vi "Autonomous Independent.vi"() -> ()   [LabVIEW 2020]
doc: "This VI is called when autonomous begins, and will automatically be terminated when autonomous ends. You can carry out timed or sensor driven robot movement independently without needing to return to the caller."
uses:
  <vilib>/Rock Robotics/WPI/Utilities/WPI_GetSetVariantRefNum.vi
  <vilib>/Rock Robotics/Network Tables/NT Read String.vi
  <vilib>/Rock Robotics/Network Tables/NT Write Numeric Array.vi
  <vilib>/Rock Robotics/WPI/RobotDrive/WPI_RobotDriveArcadeDrive_Standard(NoSaturation).vi
  2017 Swerve Code/Swerve Global Variables.vi
  Robot Global Data.vi
panel:
  out "Current Movement, for debugging":T1 {"Y Joystick Value" scale=1.0..-1.0; "X Joystick Value" scale=-1.0..1.0}
  in  "Array of robot movements":T2(array[cluster])=[{"X Joystick Value"=0.39393939393939403, "Y Joystick Value"=0.0, "Delay (sec)"=1.0, "Movement Name"="turn"}, {"X Joystick Value"=-0.3737373737373737, "Y Joystick Value"=0.0, "Delay (sec)"=1.0, "Movement Name"="turn back"}] {"Y Joystick Value" scale=1.0..-1.0; "X Joystick Value" scale=-1.0..1.0}
  # "Be sure to right-click and choose Data Operations>>Make Current Value default if you want to save the array values with the VI"
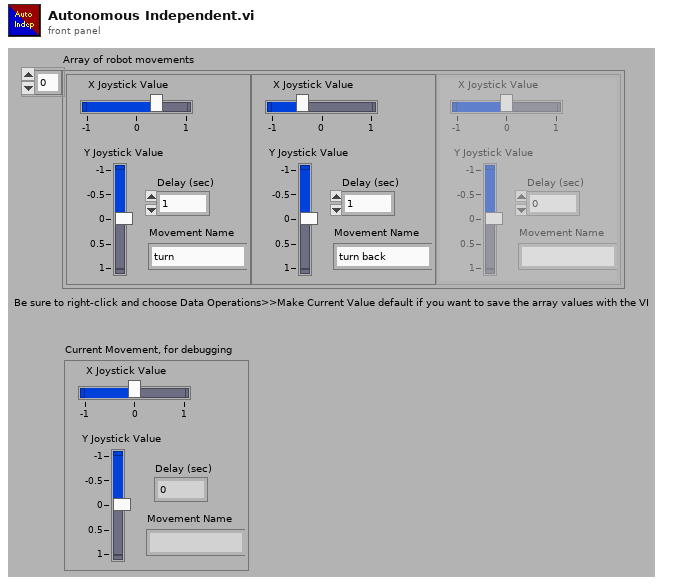
[diagram p1: front panel]
types:
  T1 = cluster{"X Joystick Value":dbl, "Y Joystick Value":dbl, "Delay (sec)":dbl, "Movement Name":string}
  T2 = cluster{"X Joystick Value":dbl, "Y Joystick Value":dbl, "Delay (sec)":dbl, "Movement Name":string}[]
  T3 = typedef "WPI_JoystickDevRef.ctl" = cluster{"Device":T4}
  T4 = typedef "WPI_JoystickDeviceEnum.ctl" = enum16{"USB 0", "USB 1", "USB 2", "USB 3", "USB 4", "USB 5"}
  T5 = typedef "WPI_RobotDriveDevRef.ctl" = cluster{"DevStatus":errorcluster, "Motors[]":T6[], "Square Inputs":bool, "Max Output":dbl}
  T6 = typedef "WPI_MotorControlDeviceRef.ctl" = cluster{"DeviceStatus":errorcluster, "Type":T7, "PWM":cluster{"PWM Channel":T8, "DeadBand":T9}, "CAN":cluster{"Device Number":u8, "SetOutput VI Ref":variant, "GetOutput VI Ref":variant, "Enable VI Ref":variant, "Disable VI Ref":variant, "Data":variant}, "Invert":bool, "DIO PWM":cluster{"PWM \"Enable\" Channel":T8, "DIOChannel":T10, "PWM Rate":dbl}}
  T7 = typedef "WPI_MotorControlType.ctl" = enum16{"PWM", "CAN", "DIO PWM"}
  T8 = typedef "FPGA_DIOPWMChannel.ctl" = enum8{"PWM 0", "PWM 1", "PWM 2", "PWM 3", "PWM 4", "PWM 5", "PWM 6", "PWM 7", "PWM 8", "PWM 9", "PWM MXP 0", "PWM MXP 1", "PWM MXP 2", "PWM MXP 3", "PWM MXP 4", "PWM MXP 5", "PWM MXP 6", "PWM MXP 7", "PWM MXP 8", "PWM MXP 9", "Invalid"}
  T9 = typedef "WPI_PWMDeadband.ctl" = cluster{"Name":string, "maxPositivePwm":i32, "minPositivePwm":i32, "centerPwm":i32, "maxNegativePwm":i32, "minNegativePwm":i32, "angularRange":u16}
  T10 = typedef "FPGA_DIOChannel.ctl" = enum8{"DIO 0", "DIO 1", "DIO 2", "DIO 3", "DIO 4", "DIO 5", "DIO 6", "DIO 7", "DIO 8", "DIO 9", "DIO MXP 0", "DIO MXP 1", "DIO MXP 2", "DIO MXP 3", "DIO MXP 4", "DIO MXP 5", "DIO MXP 6", "DIO MXP 7", "DIO MXP 8", "DIO MXP 9", "DIO MXP 10", "DIO MXP 11", "DIO MXP 12", "DIO MXP 13", "DIO MXP 14", "DIO MXP 15", "SPI Port CS1", "SPI Port CS2", "SPI Port CS3", "SPI Port MISO", "SPI Port MOSI", "Invalid"}
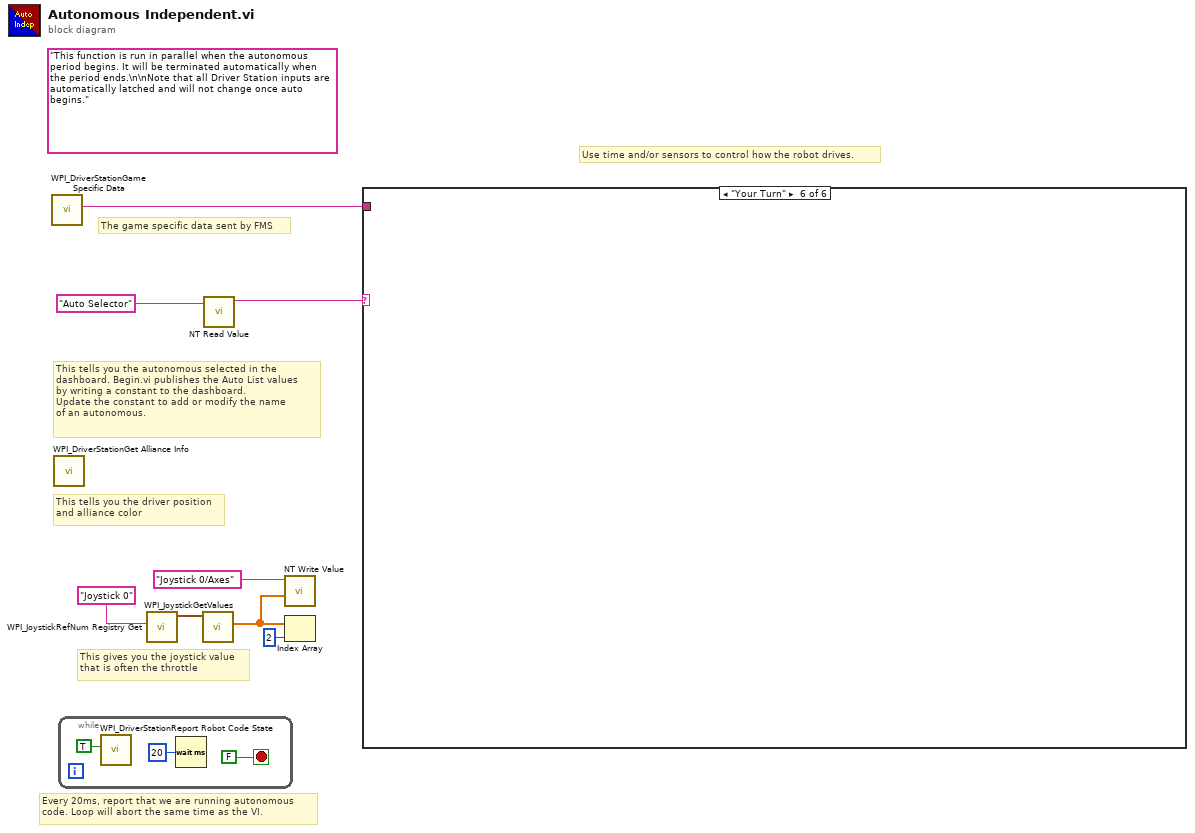
[diagram p0: block diagram]
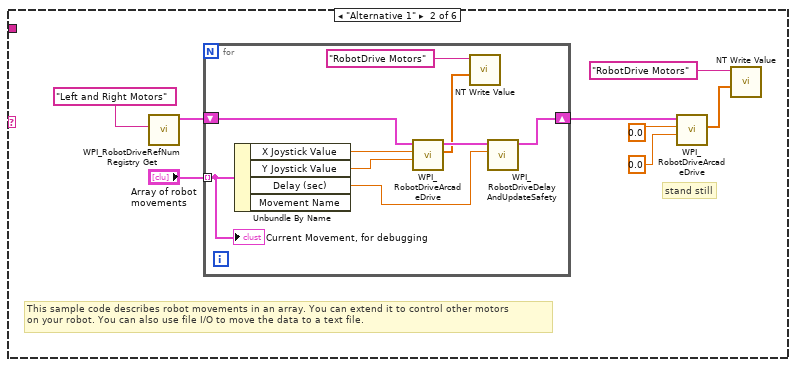
[diagram p3: hidden frame]
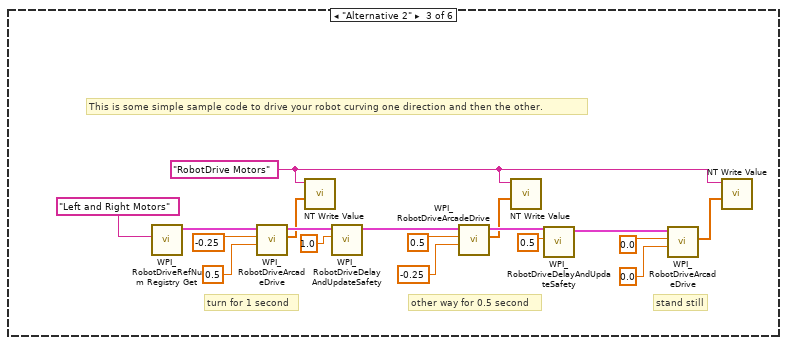
[diagram p4: hidden frame]
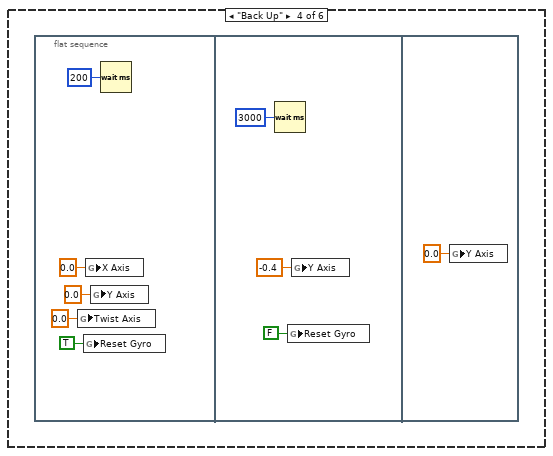
[diagram p5: hidden frame]
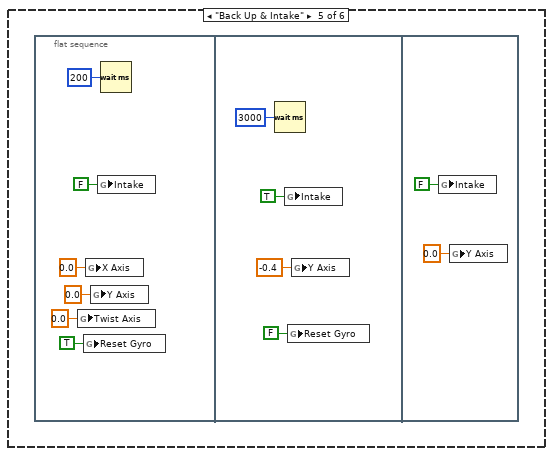
[diagram p6: hidden frame]
diagram:
  (unwired) "This function is run in parallel when the autonomous period begins. It will be terminated automatically when the period ends.\n\nNote that all Driver Station inputs are automatically latched and will not change once auto begins."
  # "The game specific data sent by FMS"
  # "This tells you the autonomous selected in the \ndashboard. Begin.vi publishes the Auto List values\nby writing a constant to the dashboard.\nUpdate the constant to add or modify the name\nof an autonomous."
  # "Every 20ms, report that we are running autonomous\ncode. Loop will abort the same time as the VI."
  # "This gives you the joystick value\nthat is often the throttle"
  # "Use time and/or sensors to control how the robot drives."
  # "This tells you the driver position\nand alliance color"
  n1 = call <vilib>:"WPI_DriverStationGame Specific Data.vi"() -> ("Game Specific Data"=w1:string)  [unwired: 11 in]
  n2 = call <vilib>:"WPI_DriverStationGet Alliance Info.vi"() -> ()  [unwired: 12 out]
  n3 = while {
    stop <- FALSE stop-if-true
    n4 = call <vilib>:"WPI_DriverStationReport Robot Code State.vi"("Autonomous"=TRUE) -> ()  [unwired: 10 in, 1 out]
    n5 = Wait (ms)(milliseconds to wait=u32 20) -> ()  [unwired: 1 out]
  }
  n6 = call <vilib>:"WPI_JoystickRefNum Registry Get.vi"("refnum name"="Joystick 0") -> ("JoystickDevRef"=w7:T3)  [unwired: 1 in, 9 out]
  n7 = call <vilib>:"WPI_JoystickGetValues.vi"("JoystickDevRef"=w7) -> ("Axes"=w3:dbl[])  [unwired: 6 in, 4 out]
  n8 = call-poly <vilib>:"NT Read Value.vi"("Name"="Auto Selector") -> ("String"=w4:string)  [unwired: 9 in, 1 out]
  n9 = call-poly <vilib>:"NT Write Value.vi"("Numeric Array"=w3, "Name"="Joystick 0/Axes") -> ()  [unwired: 9 in, 1 out]
  n10 = Index Array(array=w3, index=2) -> ()  [unwired: 1 out]
  n11 = case shown="\"Your Turn\"" w4 {
    tunnel: w1 -> [_ _ _ _ _ _]
    frame Default {
      # "You can put your main auto here, or you can right-click on the case and make any\nother frame be the default case."
      # "This is the frame that will execute if no selection is made, or if it is not recognized"
    }
    frame "Alternative 1" {
      # "stand still"
      # "This sample code describes robot movements in an array. You can extend it to control other motors\non your robot. You can also use file I/O to move the data to a text file."
      n12 = call <vilib>:"WPI_RobotDriveRefNum Registry Get.vi"("refnum name"="Left and Right Motors") -> ("RobotDriveDevRef"=w18:T5)  [unwired: 1 in, 9 out]
      n13 = for {
        shift-right: [w26] -> w13
        shift-left: w18 -> [w27]
        tunnel: "Array of robot movements" -> [w22] mode=indexing
        n14 = Unbundle By Name(w22) -> ("X Joystick Value"=w25:dbl, "Y Joystick Value"=w24:dbl, "Delay (sec)"=w23:dbl)  [unwired: 1 out]
        n15 = call-poly <vilib>:"WPI_RobotDriveArcadeDrive.vi"("Y axis value"=w24, "X axis value"=w25, "RobotDriveDevRef"=w27) -> ("Motor Values"=w20:dbl[], "RobotDriveDevRef"=w28:T5)  [unwired: 1 in, 6 out]
        n16 = call-poly <vilib>:"NT Write Value.vi"("Numeric Array"=w20, "Name"="RobotDrive Motors") -> ()  [unwired: 9 in, 1 out]
        n17 = call <vilib>:"WPI_RobotDriveDelayAndUpdateSafety.vi"("Delay (s)"=w23, "RobotDriveDevRef"=w28) -> ("RobotDriveDevRef 2"=w26:T5)  [unwired: 8 in, 1 out]
        "Current Movement, for debugging" <- w22
      }
      n18 = call-poly <vilib>:"WPI_RobotDriveArcadeDrive.vi"("Y axis value"=0.0 ("X axis value"), "X axis value"=0.0, "RobotDriveDevRef"=w13) -> ("Motor Values"=w16:dbl[])  [unwired: 1 in, 7 out]
      n19 = call-poly <vilib>:"NT Write Value.vi"("Numeric Array"=w16, "Name"="RobotDrive Motors") -> ()  [unwired: 9 in, 1 out]
    }
    frame "Alternative 2" {
      w30 = "RobotDrive Motors" ("Name")
      # "This is some simple sample code to drive your robot curving one direction and then the other."
      # "stand still"
      # "other way for 0.5 second"
      # "turn for 1 second"
      n20 = call <vilib>:"WPI_RobotDriveRefNum Registry Get.vi"("refnum name"="Left and Right Motors") -> ("RobotDriveDevRef"=w46:T5)  [unwired: 1 in, 9 out]
      n21 = call-poly <vilib>:"WPI_RobotDriveArcadeDrive.vi"("Y axis value"=0.5 ("X axis value"), "X axis value"=-0.25, "RobotDriveDevRef"=w46) -> ("Motor Values"=w29:dbl[], "RobotDriveDevRef"=w39:T5)  [unwired: 1 in, 6 out]
      n22 = call-poly <vilib>:"NT Write Value.vi"("Numeric Array"=w29, "Name"=w30) -> ()  [unwired: 9 in, 1 out]
      n23 = call <vilib>:"WPI_RobotDriveDelayAndUpdateSafety.vi"("Delay (s)"=1.0, "RobotDriveDevRef"=w39) -> ("RobotDriveDevRef 2"=w40:T5)  [unwired: 8 in, 1 out]
      n24 = call-poly <vilib>:"WPI_RobotDriveArcadeDrive.vi"("Y axis value"=-0.25 ("X axis value"), "X axis value"=0.5, "RobotDriveDevRef"=w40) -> ("Motor Values"=w31:dbl[], "RobotDriveDevRef"=w41:T5)  [unwired: 1 in, 6 out]
      n25 = call-poly <vilib>:"NT Write Value.vi"("Numeric Array"=w31, "Name"=w30) -> ()  [unwired: 9 in, 1 out]
      n26 = call <vilib>:"WPI_RobotDriveDelayAndUpdateSafety.vi"("Delay (s)"=0.5, "RobotDriveDevRef"=w41) -> ("RobotDriveDevRef 2"=w42:T5)  [unwired: 8 in, 1 out]
      n27 = call-poly <vilib>:"WPI_RobotDriveArcadeDrive.vi"("Y axis value"=0.0 ("X axis value"), "X axis value"=0.0, "RobotDriveDevRef"=w42) -> ("Motor Values"=w32:dbl[])  [unwired: 1 in, 7 out]
      n28 = call-poly <vilib>:"NT Write Value.vi"("Numeric Array"=w32, "Name"=w30) -> ()  [unwired: 9 in, 1 out]
    }
    frame "Back Up" {
      n29 = flat-sequence {
        frame #0 {
          n30 = global write "Swerve Global Variables.vi" "Twist Axis"(0.0 ("Twist Axis")) -> ()
          n31 = global write "Swerve Global Variables.vi" "Reset Gyro"(TRUE ("Reset Gyro")) -> ()
          n32 = global write "Swerve Global Variables.vi" "X Axis"(0.0 ("X Axis")) -> ()
          n33 = global write "Swerve Global Variables.vi" "Y Axis"(0.0 ("Y Axis")) -> ()
          n34 = Wait (ms)(milliseconds to wait=u32 200) -> ()  [unwired: 1 out]
        }
        frame #1 {
          n35 = Wait (ms)(milliseconds to wait=u32 3000) -> ()  [unwired: 1 out]
          n36 = global write "Swerve Global Variables.vi" "Reset Gyro"(FALSE ("Reset Gyro")) -> ()
          n37 = global write "Swerve Global Variables.vi" "Y Axis"(-0.4 ("Y Axis")) -> ()
        }
        frame #2 {
          n38 = global write "Swerve Global Variables.vi" "Y Axis"(0.0 ("Y Axis")) -> ()
        }
      }
    }
    frame "Back Up & Intake" {
      n39 = flat-sequence {
        frame #0 {
          n40 = global write "Swerve Global Variables.vi" "Twist Axis"(0.0 ("Twist Axis")) -> ()
          n41 = global write "Swerve Global Variables.vi" "Reset Gyro"(TRUE ("Reset Gyro")) -> ()
          n42 = global write "Swerve Global Variables.vi" "X Axis"(0.0 ("X Axis")) -> ()
          n43 = global write "Swerve Global Variables.vi" "Y Axis"(0.0 ("Y Axis")) -> ()
          n44 = global write "Robot Global Data.vi" "Intake"(FALSE ("Intake")) -> ()
          n45 = Wait (ms)(milliseconds to wait=u32 200) -> ()  [unwired: 1 out]
        }
        frame #1 {
          n46 = Wait (ms)(milliseconds to wait=u32 3000) -> ()  [unwired: 1 out]
          n47 = global write "Robot Global Data.vi" "Intake"(TRUE ("Intake")) -> ()
          n48 = global write "Swerve Global Variables.vi" "Reset Gyro"(FALSE ("Reset Gyro")) -> ()
          n49 = global write "Swerve Global Variables.vi" "Y Axis"(-0.4 ("Y Axis")) -> ()
        }
        frame #2 {
          n50 = global write "Robot Global Data.vi" "Intake"(FALSE ("Intake")) -> ()
          n51 = global write "Swerve Global Variables.vi" "Y Axis"(0.0 ("Y Axis")) -> ()
        }
      }
    }
    frame "Your Turn" {
    }
  }
